vi "Test Add UID To Parent List.vi"(8 "error in (no error)":errorcluster) -> (0 "error out":errorcluster)   [LabVIEW 2017, in "Unit Tests.lvlib"]
uses:
  Unit Tests.lvlib
  <vilib>/addons/_JKI Toolkits/Caraya/classes/Test/Test.lvclass
  <vilib>/addons/_JKI Toolkits/Caraya/classes/Assert/Assert.lvclass
  source/Browser Core/Server Classes/Base Tree/Base Tree.lvclass
  source/Browser Core/Node Classes/Generic Node/Generic Node.lvclass
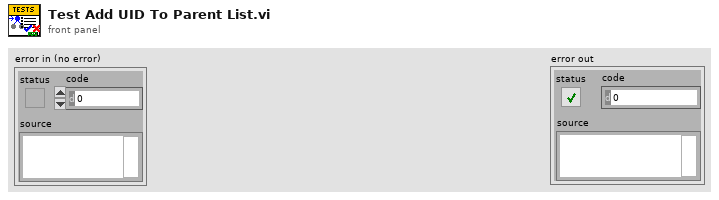
[diagram p1: front panel]
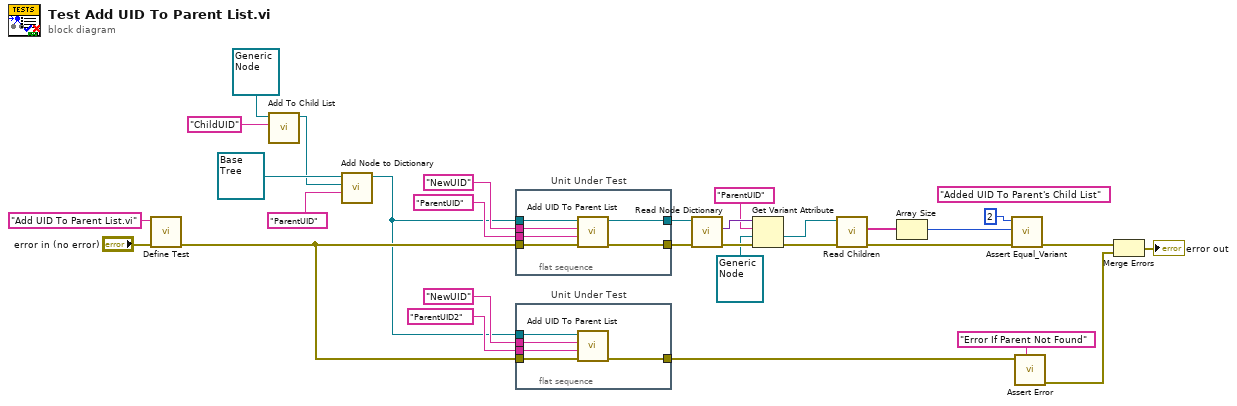
[diagram p0: block diagram]
diagram:
  (unwired) "Added UID To Parent's Child List" ("Label")
  n1 = call <vilib>:"Define Test.vi"("error in (no error)"="error in (no error)", "Label (VI Title)"="Add UID To Parent List.vi") -> ("error out"=w17:errorcluster)  [unwired: 9 in]
  n2 = call-dynamic "Add To Child List.vi"("Child ID"="ChildUID", "Generic Node in"=refnum<class "Generic Node.lvclass"> refnum ("New Node")) -> ("Generic Node out"=w9:refnum<class "Generic Node.lvclass">)  [unwired: 9 in]
  n3 = call "Add Node to Dictionary.vi"("UID"="ParentUID", "New Node"=w9, "Base Tree in"=refnum<class "Base Tree.lvclass"> refnum ("Browser Core.lvlib:Base Tree.lvclass")) -> ("Base Tree out"=w16:refnum<class "Base Tree.lvclass">)  [unwired: 8 in]
  n4 = flat-sequence "Unit Under Test" {
    tunnel: w17 -> [w36]
    tunnel: w16 -> [w35]
    tunnel: "ParentUID" -> [w34]
    tunnel: "NewUID" -> [w33]
    tunnel: [w32] -> w8
    tunnel: [w31] -> w7
    frame #0 {
      n5 = call "Add UID To Parent List.vi"("Base Tree in"=w35, "UID"=w33, "Parent"=w34, "error in (no error)"=w36) -> ("Base Tree out"=w31:refnum<class "Base Tree.lvclass">, "error out"=w32:errorcluster)  [unwired: 5 in]
    }
  }
  n6 = flat-sequence "Unit Under Test" {
    tunnel: w17 -> [w41]
    tunnel: w16 -> [w40]
    tunnel: "ParentUID2" -> [w39]
    tunnel: "NewUID" -> [w38]
    tunnel: [w37] -> w15
    frame #0 {
      n7 = call "Add UID To Parent List.vi"("Base Tree in"=w40, "UID"=w38, "Parent"=w39, "error in (no error)"=w41) -> ("error out"=w37:errorcluster)  [unwired: 5 in, 1 out]
    }
  }
  n8 = call "Read Node Dictionary.vi"("error in (no error)"=w8, "Base Tree in"=w7) -> ("error out"=w6:errorcluster, "Node Dictionary"=w5:variant)  [unwired: 7 in, 1 out]
  n9 = Get Variant Attribute(Variant=w5, name="ParentUID", default value (empty Variant)=refnum<class "Generic Node.lvclass"> refnum ("New Node"), error in=w6) -> (value=w1:refnum<class "Generic Node.lvclass">, error out=w3:errorcluster)  [unwired: 2 out]
  n10 = call "Read Children.vi"("error in (no error)"=w3, "Generic Node in"=w1) -> ("error out"=w13:errorcluster, "Children"=w14:string[])  [unwired: 7 in, 1 out]
  n11 = Array Size(array=w14) -> (size(s)=w11:i32)
  n12 = call <vilib>:"Assert Equal_Variant.vi"("error in (no error)"=w13, "Y"=w11, "X"=2 ("size(s)")) -> ("error out"=w12:errorcluster)  [unwired: 8 in]
  n13 = call <vilib>:"Assert Error.vi"("Label"="Error If Parent Not Found", "Error?"=w15) -> ("error out"=w29:errorcluster)  [unwired: 9 in]
  n14 = Merge Errors(w12, w29) -> (→"error out":errorcluster)
